vi "P4CMDSub Fstat.vi"(8 "error in (no error)":errorcluster, 10 "files":path[](array[path]), 11 "source control reference in":T1) -> (0 "error out":errorcluster, 1 "files status":T2[](array[typedef]), 2 "fstat output":string, 3 "source control reference out":T1)   [LabVIEW 2017, in "NI_SCC_P4CMD.lvlib"]
uses:
  <vilib>/SourceControl/Providers/P4CMD/NI_SCC_P4CMD.lvlib
  <vilib>/SourceControl/Providers/P4CMD/P4CMD SCC File Status.ctl
  <vilib>/SourceControl/sccapi/SCCAPI Refnum.ctl
  <vilib>/SourceControl/Providers/P4CMD/P4CMD Operations.ctl
  <vilib>/SourceControl/sccapi/NI_SCC.lvlib
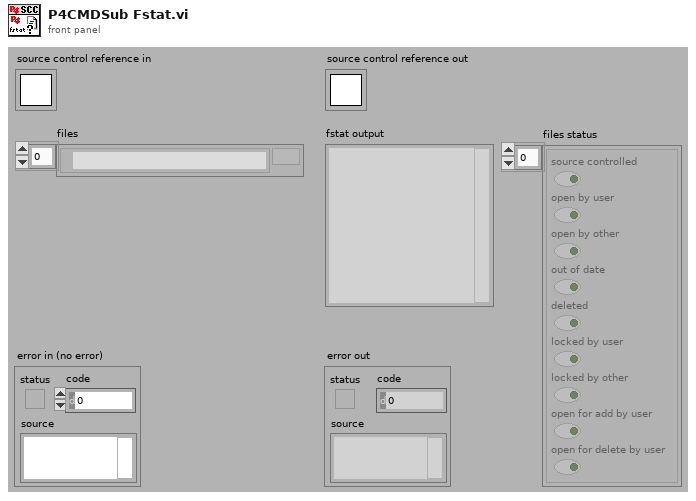
[diagram p1: front panel]
types:
  T1 = typedef "NI_SCC.lvlib/SCCAPI Refnum.ctl" = refnum<k1>
  T2 = typedef "NI_SCC_P4CMD.lvlib/P4CMD SCC File Status.ctl" = cluster{"source controlled":bool, "open by user":bool, "open by other":bool, "out of date":bool, "deleted":bool, "locked by user":bool, "locked by other":bool, "open for add by user":bool, "open for delete by user":bool}
  T3 = typedef "NI_SCC_P4CMD.lvlib/P4CMD Operations.ctl" = enum16{"get all clients", "get all users", "describe changelist", "sync from depot", "open for edit", "submit to depot", "revert", "add to depot", "remove from depot", "print files revisions", "compare client file", "print depot file contents", "list opened files", "get file info", "lock files", "edit changelist spec", "info", "set variables"}
  T4 = enum32{"invalid OS target", "Mac OS", "Windows 3.1", "Windows 95/NT", "Solaris 1", "Solaris 2", "HP-UX", "PowerMAX", "Linux", "Irix", "Rhapsody", "BeOS", "AIX", "OSF1", "VxWorks", "PharLap", "Carbon", "RTX", "Windows x64", "Linux x64", "Mac OS X x64"}
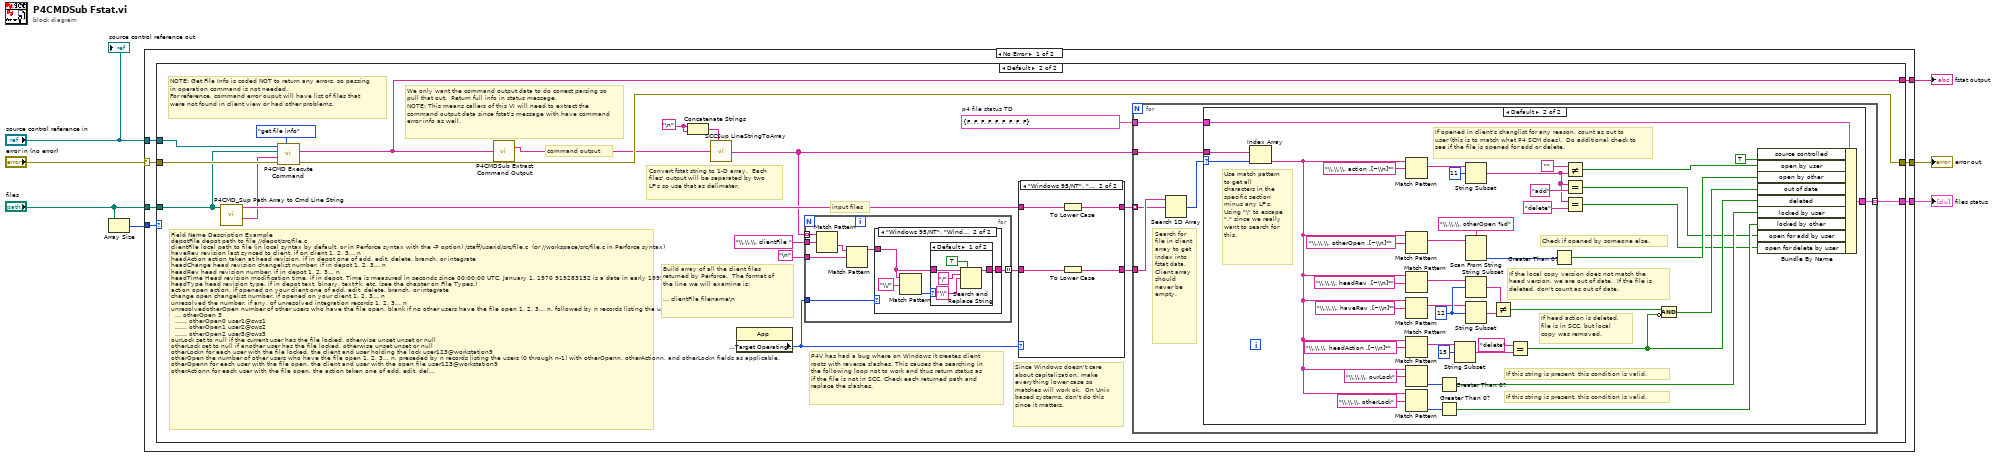
[diagram p0: block diagram]
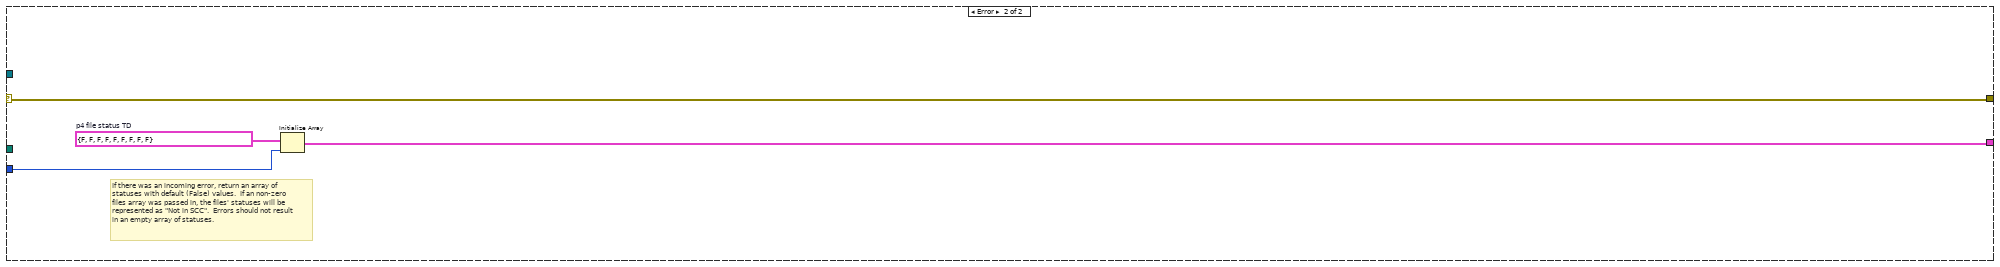
[diagram p7: hidden frame]
diagram:
  n1 = Array Size(array="files") -> (size(s)=w1:i32)
  n2 = case shown="No Error" "error in (no error)" {
    selector: "error in (no error)" -> [w14 w112]
    tunnel: "files" -> [w9 _]
    tunnel: [w13 w112] -> w7
    tunnel: [w12 w111] -> w4
    tunnel: [w11 _] -> w5
    tunnel: "source control reference in" -> [w10 _]
    tunnel: w1 -> [w8 w110]
    frame No Error {
      n3 = case shown="Default" w8 {
        tunnel: w14 -> [w15 w35]
        tunnel: [w15 w32] -> w13
        tunnel: [_ w31] -> w12
        tunnel: [_ w18] -> w11
        tunnel: w10 -> [_ w29]
        tunnel: w9 -> [_ w28]
        frame 0 {
          # "If there were no files in array, don't do anything.  Returning an empty status array is not preferred, but have not choice since there were no files with which to work with."
        }
        frame Default {
          w21 = T2 {"source controlled"=FALSE, "open by user"=FALSE, "open by other"=FALSE, "out of date"=FALSE, "deleted"=FALSE, "locked by user"=FALSE, "locked by other"=FALSE, "open for add by user"=FALSE, "open for delete by user"=FALSE}  # p4 file status TD
          w27 = "\n"
          # "P4V has had a bug where on Windows it creates client roots with reverse slashes. This causes the searching in the following loop not to work and thus return status as if the file is not in SCC. Check each returned path and replace the slashes."
          # "We only want the command output data to do correct parsing so pull that out.  Return full info in status message.\nNOTE: This means callers of this VI will need to extract the command output data since fstat's message with have command error info as well."
          # "input files"
          # "Since Windows doesn't care about capitalization, make everything lower case so matches will work ok.  On Unix based systems, don't do this since it matters."
          # "Convert fstat string to 1-D array.  Each files' output will be separated by two LF's so use that as delimeter."
          # "Build array of all the client files returned by Perforce.  The format of the line we will examine is:\n\n... clientFile filename\\n"
          # "NOTE: Get File Info is coded NOT to return any errors, so passing in operation command is not needed.\nFor reference, command error ouput will have list of files that were not found in client view or had other problems."
          # "command output"
          # "Field Name\tDescription\tExample\ndepotFile\tdepot path to file\t//depot/src/file.c\nclientFile\tlocal path to file (in local syntax by default, or in Perforce syntax with the -P option)\t/staff/userid/src/file.c\t\t(or //workspace/src/file.c in Perforce syntax)\nhaveRev\trevision last synced to client, if on client\t1, 2, 3... n\nheadAction\taction taken at head revision, if in depot\tone of add, edit, delete, branch, or integrate\nheadChange\thead revision changelist number, if in depot\t1, 2, 3... n\nheadRev\thead revision number, if in depot\t1, 2, 3... n\nheadTime\tHead revision modification time, if in depot. Time is measured in seconds since 00:00:00 UTC, January 1, 1970\t919283152 is a date in early 1999\nheadType\thead revision type, if in depot\ttext, binary, text+k, etc. (see the chapter on File Types.)\naction\topen action, if opened on your client\tone of add, edit, delete, branch, or integrate\nchange\topen changelist number, if opened on your client\t1, 2, 3... n\nunresolved\tthe number, if any, of unresolved integration records\t1, 2, 3... n\nunresolvedotherOpen\tnumber of other users who have the file open, blank if no other users have the file open\t1, 2, 3... n, followed by n records listing the users (0 through n-1):\n\t\t... otherOpen 3\n\t\t...... otherOpen0 user1@cws1\n\t\t...... otherOpen1 user2@cws2\n\t\t...... otherOpen2 user3@cws3\nourLock\tset to null if the current user has the file locked, otherwise unset\tunset or null\notherLock\tset to null if another user has the file locked, otherwise unset\tunset or null\notherLockn\tfor each user with the file locked, the client and user holding the lock\tuser123@workstation9\notherOpen\tthe number of other users who have the file open\t1, 2, 3... n, preceded by n records listing the users (0 through n-1) with otherOpenn, otherActionn, and otherLockn fields as applicable.\notherOpenn\tfor each user with the file open, the client and user with the open file\tuser123@workstation9\notherActionn\tfor each user with the file open, the action taken\tone of add, edit, delete, branch, or integrate\nfileSize\tfile length in bytes (requires -l option, may be expensive to compute)\t63488"
          n4 = call <vilib>:"P4CMD_Sup Path Array to Cmd Line String.vi"("files"=w28) -> ("string output"=w30:string, "converted file strings"=w33:string[])  [unwired: 9 in]
          n5 = call <vilib>:"P4CMD Execute Command.vi"("p4 operation"=P4CMD_Operations."get file info", "error in (no error)"=w35, "input string"=w30, "files"=w28, "source control reference in"=w29) -> ("error out"=w32:errorcluster, "command information"=w18:string)  [unwired: 4 in, 1 out]
          n6 = call <vilib>:"P4CMDSub Extract Command Output.vi"("bundled message"=w18) -> ("command output"=w17:string)  [unwired: 13 in, 1 out]
          n7 = Concatenate Strings(w27, w27) -> (w19:string)
          n8 = call <vilib>:"SCCSup LineStringToArray.vi"("delimiter (Tab)"=w19, "line string"=w17) -> ("line array"=w20:string[])  [unwired: 7 in]
          n9 = property class="App"() -> ("Application:Target Operating System"=w16:T4)  [unwired: 2 in, 2 out]
          n10 = for {
            tunnel: "\\.\\.\\. clientFile " ("regular expression") -> [w48]
            tunnel: "\n" -> [w45]
            tunnel: w20 -> [w46] mode=indexing
            tunnel: [w43] -> w24 mode=indexing
            tunnel: w16 -> [w42]
            n11 = Match Pattern(string=w46, regular expression=w48) -> (after substring=w47:string)  [unwired: 1 in, 3 out]
            n12 = Match Pattern(string=w47, regular expression=w45) -> (before substring=w44:string)  [unwired: 1 in, 3 out]
            n13 = case shown="\"Windows 95/NT\", \"Windows x64\"" w42 {
              tunnel: [w49 w51] -> w43
              tunnel: w44 -> [w49 w50]
              frame "invalid OS target", Default {
              }
              frame "Windows 95/NT", "Windows x64" {
                n14 = Match Pattern(string=w50, regular expression="\\/") -> (offset past match=w52:i32)  [unwired: 1 in, 3 out]
                n15 = case shown="Default" w52 {
                  tunnel: w50 -> [w58 w59]
                  tunnel: [w54 w59] -> w51
                  frame Default {
                    n16 = Search and Replace String(replace all?=TRUE ("replace all? (F)"), input string=w58, search string="/" ("regular expression"), replace string="\\" ("regular expression")) -> (result string=w54:string)  [unwired: 4 in, 3 out]
                  }
                  frame -1 {
                  }
                }
              }
            }
          }
          n17 = case shown="\"Windows 95/NT\", \"Windows x64\"" w16 {
            tunnel: w33 -> [w37 w41]
            tunnel: w24 -> [w36 w40]
            tunnel: [w37 w39] -> w23
            tunnel: [w36 w38] -> w22
            frame Default {
            }
            frame "Windows 95/NT", "Windows x64" {
              n18 = To Lower Case(string=w41) -> (all lower case string=w39:string[])
              n19 = To Lower Case(string=w40) -> (all lower case string=w38:string[])
            }
          }
          n20 = for {
            tunnel: w20 -> [w63]
            tunnel: w23 -> [w61] mode=indexing
            tunnel: w21 -> [w65]
            tunnel: [w64] -> w31 mode=indexing
            tunnel: w22 -> [w62]
            # "Search for file in client array to get index into fstat data.  Client array should never be empty."
            n21 = Search 1D Array(1D array=w62, element=w61) -> (index of element=w60:i32)  [unwired: 1 in]
            n22 = case shown="Default" w60 {
              selector: w60 -> [_ w87]
              tunnel: w65 -> [w66 w86]
              tunnel: [w66 w85] -> w64
              tunnel: w63 -> [_ w88]
              frame -1 {
                # "If file was not found in client files list array, treat as not in source control.  This probably means it was not found in SCC under this client.  The file may be under SCC under another client, but will treat as not in SCC for this one. Default values from constant are passed through (source controlled bit will be false)."
              }
              frame Default {
                w93 = 12
                # "If this string is present, this condition is valid."
                # "If this string is present, this condition is valid."
                # "If head action is deleted, file is in SCC, but local copy was removed."
                # "Check if opened by someone else."
                # "If opened in client's changlist for any reason, count as out to user (this is to match what P4 SCM does).  Do additional check to see if the file is opened for add or delete."
                # "Use match pattern to get all characters in the specific section minus any LF's.  Using \"\\\" to escape \".\" since we really want to search for this."
                # "If the local copy version does not match the head version, we are out of date.  If the file is deleted, don't count as out of date."
                n23 = Index Array(array=w88, index=w87) -> (element=w79:string)
                n24 = Match Pattern(string=w79, regular expression="\\.\\.\\. action .[~\\n]*") -> (match substring=w103:string)  [unwired: 1 in, 3 out]
                n25 = Match Pattern(string=w79, regular expression="\\.\\.\\. otherOpen .[~\\n]*") -> (match substring=w100:string)  [unwired: 1 in, 3 out]
                n26 = Match Pattern(string=w79, regular expression="\\.\\.\\. headRev .[~\\n]*") -> (match substring=w94:string)  [unwired: 1 in, 3 out]
                n27 = Match Pattern(string=w79, regular expression="\\.\\.\\. haveRev .[~\\n]*") -> (match substring=w90:string)  [unwired: 1 in, 3 out]
                n28 = Match Pattern(string=w79, regular expression="\\.\\.\\. headAction .[~\\n]*") -> (match substring=w96:string)  [unwired: 1 in, 3 out]
                n29 = Match Pattern(string=w79, regular expression="\\.\\.\\. ourLock") -> (offset past match=w78:i32)  [unwired: 1 in, 3 out]
                n30 = Match Pattern(string=w79, regular expression="\\.\\.\\. otherLock") -> (offset past match=w76:i32)  [unwired: 1 in, 3 out]
                n31 = Greater Than 0?(x=w78) -> (x > 0?=w77:bool)
                n32 = Greater Than 0?(x=w76) -> (x > 0?=w75:bool)
                n33 = String Subset(string=w96, offset (0)=15) -> (substring=w106:string)  [unwired: 1 in]
                n34 = String Subset(string=w103, offset (0)=11) -> (substring=w69:string)  [unwired: 1 in]
                n35 = Scan From String(format string="\\.\\.\\. otherOpen %d", input string=w100) -> (output 1=w97:i32)  [unwired: 3 in, 3 out]
                n36 = String Subset(string=w94, offset (0)=w93) -> (substring=w92:string)  [unwired: 1 in]
                n37 = String Subset(string=w90, offset (0)=w93) -> (substring=w89:string)  [unwired: 1 in]
                n38 = Not Equal?(x=w92, y=w89) -> (x != y?=w74:bool)
                n39 = Equal?(x="delete", y=w106) -> (x = y?=w72:bool)
                n40 = Greater Than 0?(x=w97) -> (x > 0?=w82:bool)
                n41 = Not Equal?(x="", y=w69) -> (x != y?=w83:bool)
                n42 = Equal?(x=w69, y="add") -> (x = y?=w68:bool)
                n43 = Equal?(x=w69, y="delete") -> (x = y?=w67:bool)
                n44 = Compound Arithmetic op=AND(w74, invert w72) -> (w73:bool)
                n45 = Bundle By Name(cluster=w86, "source controlled"=TRUE, "open by user"=w83, "open by other"=w82, "out of date"=w73, "deleted"=w72, "locked by user"=w77, "locked by other"=w75, "open for add by user"=w68, "open for delete by user"=w67) -> (w85:T2)
              }
            }
          }
        }
      }
    }
    frame Error {
      w109 = T2 {"source controlled"=FALSE, "open by user"=FALSE, "open by other"=FALSE, "out of date"=FALSE, "deleted"=FALSE, "locked by user"=FALSE, "locked by other"=FALSE, "open for add by user"=FALSE, "open for delete by user"=FALSE}  # p4 file status TD
      # "If there was an incoming error, return an array of statuses with default (False) values.  If an non-zero files array was passed in, the files' statuses will be represented as \"Not in SCC\".  Errors should not result in an empty array of statuses."
      n46 = Initialize Array(w109, w110) -> (w111:T2[])
    }
  }
  "error out" <- w7
  "files status" <- w4
  "fstat output" <- w5
  "source control reference out" <- "source control reference in"
